vi "Enable Logic Analyzer Display.vi"(8 "error in (no error)":errorcluster, 10 "Enable Display (F: Disable)":bool, 11 "VISA resource name":refnum<visa-resource-name>) -> (0 "error out":errorcluster, 3 "VISA resource name out":refnum<visa-resource-name>)   [LabVIEW 2015, in "RIGOL DS1000 Series.lvlib"]
doc: "Enables or disables logic analyzer display.\n\nNote:\nThis VI is only valid for DS1052D and DS1102D."
uses:
  RIGOL DS1000 Series.lvlib
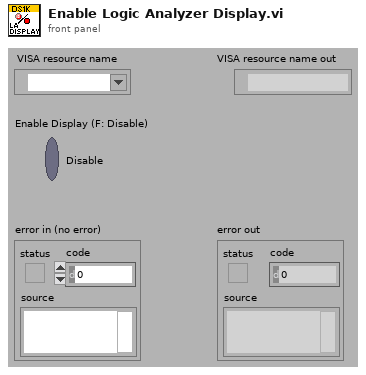
[diagram p1: front panel]
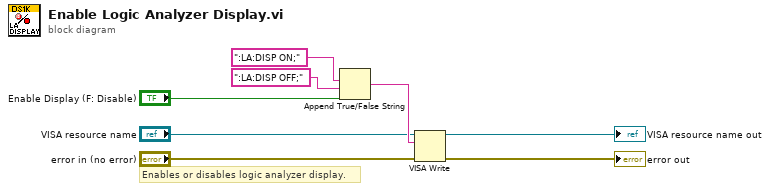
[diagram p0: block diagram]
diagram:
  # "Enables or disables logic analyzer display."
  n1 = Append True/False String(1:"Enable Display (F: Disable)", 2:":LA:DISP OFF;", 3:":LA:DISP ON;") -> (0:w5:string)  [unwired: 1 out]
  n2 = VISA Write(VISA resource name="VISA resource name", write buffer=w5, error in (no error)="error in (no error)") -> (VISA resource name out=→"VISA resource name out":refnum<visa-resource-name>, error out=→"error out":errorcluster)  [unwired: 1 out]
